vi "SVFA FFT Spectrum (Real-Im) (1 Ch).vi"(0 "scaled signal [EU]":waveform(dbl), 2 "window":T9=1 items=["None"=0, "Hanning"=1, "Hamming"=2, "Blackman-Harris"=3, "Exact Blackman"=4, "Blackman"=5, "Flat Top"=6, "4 Term B-Harris "=7, "7 Term B-Harris"=8, "Low Sidelobe"=9, "Force"=64, "Exponential"=65, "Blackman Nuttall"=11, "Triangle"=30, "Bartlett-Hanning"=31, "Bohman"=32, "Parzen"=33, "Welch"=34, "Kaiser"=60, "Dolph-Chebyshev"=61, "Gaussian"=62], 5 "error in (no error)":errorcluster, 7 "averaging parameters":T7={"averaging mode"=enum."No averaging", "weighting mode"=enum."Exponential", "number of averages"=10, "linear mode"=enum."One shot"} {"number of averages" min=1 step=1}, 9 "restart averaging (F)":bool) -> (11 "averaging done":bool, 13 "averages completed":dbl, 14 "real part [EU rms]":cluster{"f0":dbl, "df":dbl, "real part":dbl[]} {"real part" format="%.2f"; "df" format="%.2f"; "f0" format="%.2f"}, 16 "imaginary part [EU rms]":T8 {"imaginary part" format="%.2f"; "df" format="%.2f"; "f0" format="%.2f"}, 17 "unit label":string, 18 "spectrum info":T1={"channel name"="", "description"="", "x-axis units"=0, "spectral info"={"spectrum type"=enum."Power [Magnitude^2]", "linear/dB"=enum."linear", "window"=0, "window size"=0, "FFT size"=0}, "engineering units"=0, "custom label"="", "dB reference [EU]"=0.0, "peak units"=enum."rms", "weighting filter"=0, "spectral density?"=FALSE, "unit label"="", "spectrum skewed?"=FALSE, "complimentary spectrum units"=enum."none"} {"x-axis units" items=["Time (s)"=0, "Frequency-CB (Hz)"=1, "Frequency-CPB (Hz)"=1248, "Frequency-Arbitrary (Hz)"=2357, "Quefrency (s)"=2, "Revolutions (rev)"=3, "Order"=4, "Speed (RPM)"=11, "Speed (rad/s)"=21, "Index"=65535]; "weighting filter" items=["Linear", "A-weighting", "B-weighting", "C-weighting", "ITU-R 468-4", "Dolby", "CCITT", "C-message", "Wb", "Wc", "Wd", "We", "Wf", "Wh", "Wj", "Wk", "Wm", "AES17 20 kHz lowpass", "AES17 40 kHz lowpass", "AES17 20 kHz highpass", "AES17 40 kHz highpass"]; "dB reference [EU]" format="%.2f"; "engineering units" items=["custom..."=0, "V"=1, "A"=21, "C"=30, "pC"=31, "s"=32, "-"=29, "Pa"=2, "N"=20, "g"=3, "m/s^2"=4, "m/s"=5, "m"=6, "mm/s"=12, "mm"=13, "micron/s"=14, "micron"=15, "in/s^2"=7, "in/s"=8, "in"=9, "mil/s"=10, "mil"=11, "rad/s^2"=16, "rad/s"=17, "rad"=18, "deg/s^2"=26, "deg/s"=27, "deg"=28, "RPM"=22, "cycle/s^2"=23, "Hz"=24, "cycle"=25, "strain"=19]; "spectral info"."window" items=["None "=0, "Hanning"=1, "Hamming"=2, "Blackman-Harris"=3, "Exact Blackman"=4, "Blackman"=5, "Flat Top"=6, "4 Term B-Harris "=7, "7 Term B-Harris"=8, "Low Sidelobe"=9, "Force - Exponential"=10, "Gaussian"=62]}, 19 "error out":errorcluster)   [LabVIEW 2017]
doc: "Computes the Fast Fourier Transform (FFT) spectrum of <B>scaled signal [EU]</B>. This VI returns FFT results as the real and imaginary parts, or the first and second elements of the ordered pairs, of the FFT spectrum. Wire data to the <B>scaled signal [EU]</B> input to determine the polymorphic instance to use or manually select the instance."
uses:
  <vilib>/addons/_NISVFA/_Shared subVIs/Controls/svc_Window.ctl
  <vilib>/addons/_NISVFA/_Shared subVIs/Controls/svc_Spectrum Info.ctl
  <vilib>/addons/_NISVFA/_Shared subVIs/Controls/svc_X-Axis Units.ctl
  <vilib>/addons/_NISVFA/_Shared subVIs/Controls/svc_Spectrum Type.ctl
  <vilib>/addons/_NISVFA/_Shared subVIs/Controls/svc_Engineering Units Text Ring.ctl
  <vilib>/addons/_NISVFA/_Shared subVIs/Controls/svc_Weighting Filter Text Ring.ctl
  <vilib>/addons/_NISVFA/_Shared subVIs/Controls/svc_Complimentary Spectrum Units.ctl
  <vilib>/Analysis/2dsp.llb/Real FFT.vi
  <vilib>/Analysis/2dsp.llb/Power Spectrum (DBL).vi
  <vilib>/addons/_NISVFA/_Shared subVIs/Windowing/svfa_Scaled Time Domain Window (Array).vi
  <vilib>/addons/_NISVFA/_Shared subVIs/Common/svc_Get SV Channel Info.vi
  <vilib>/addons/_NISVFA/_Shared subVIs/Common/svc_Spectrum Units.vi
  <vilib>/addons/_NISVFA/_Shared subVIs/Spectrum Averaging/svfa_No Average Array (complex).vi
  <vilib>/addons/_NISVFA/_Shared subVIs/Spectrum Averaging/svfa_Average Array (complex).vi
  <vilib>/addons/_NISVFA/_Shared subVIs/Spectrum Averaging/svfa_No Average Array (real).vi
  <vilib>/addons/_NISVFA/_Shared subVIs/Spectrum Averaging/svfa_Average Array (real).vi
  <vilib>/addons/_NISVFA/_Shared subVIs/Spectrum Averaging/svfa_Peak Hold Array.vi
  <vilib>/Analysis/4window.llb/Force Window.vi
  <vilib>/Analysis/4window.llb/Force Window (DBL).vi
  <vilib>/Analysis/4window.llb/Exponential Window.vi
  <vilib>/Analysis/4window.llb/Exponential Window (DBL).vi
  <vilib>/Utility/error.llb/Error Cluster From Error Code.vi
  <vilib>/Analysis/0measdsp.llb/Scaled Time Domain Window.vi
  <vilib>/Analysis/0measdsp.llb/Scaled Time Domain Window (DBL).vi
  <vilib>/addons/_NISVFA/_Spectrum Processing/subVIs/svfa_Spectrum Info Window to windowTd Type Def.vi
  <vilib>/addons/_NISVFA/_Shared subVIs/Common/svc_Window Parameters.vi
  <vilib>/addons/_NISVFA/_Shared subVIs/Common/svc_Get Window Info.vi
  <vilib>/addons/_NISVFA/_Shared subVIs/Common/svc_Get Weighting Enum and Labels.vi
  <vilib>/addons/_NISVFA/_Shared subVIs/Common/svc_Unit Label Lexical Class.vi
  <vilib>/addons/_NISVFA/_Shared subVIs/Common/svc_Engineering Units to Unit Label.vi
  <vilib>/addons/_NISVFA/_Shared subVIs/Common/svc_Format Value (DBL).vi
  <vilib>/addons/_NISVFA/_Shared subVIs/Common/svc_Channel Info to Spectrum Info.vi
  <vilib>/addons/_NISVFA/_Shared subVIs/Common/svc_Unit Label to Engineering Units.vi
  <vilib>/Analysis/NI_AALPro.lvlib
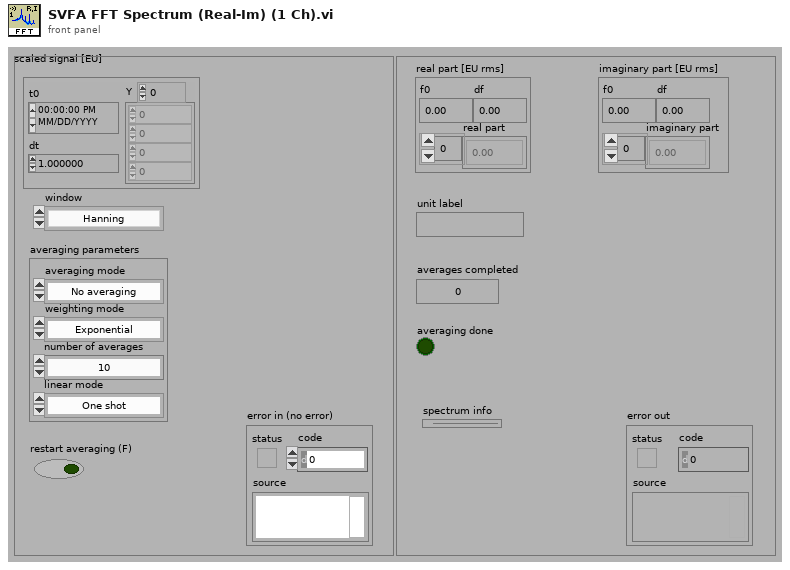
[diagram p1: front panel]
types:
  T1 = typedef "svc_Spectrum Info.ctl" = cluster{"channel name":string, "description":string, "x-axis units":T2, "spectral info":cluster{"spectrum type":T3, "linear/dB":enum16{"linear", "dB"}, "window":u16, "window size":i32, "FFT size":i32}, "engineering units":T4, "custom label":string, "dB reference [EU]":dbl, "peak units":enum16{"rms", "peak", "peak-peak"}, "weighting filter":T5, "spectral density?":bool, "unit label":string, "spectrum skewed?":bool, "complimentary spectrum units":T6}
  T2 = typedef "svc_X-Axis Units.ctl" = u16
  T3 = typedef "svc_Spectrum Type.ctl" = enum16{"FFT Spectrum [complex]", "Amplitude [Magnitude]", "Power [Magnitude^2]", "Cross Spectrum [complex]", "Frequency Response [Complex]"}
  T4 = typedef "svc_Engineering Units Text Ring.ctl" = u16
  T5 = typedef "svc_Weighting Filter Text Ring.ctl" = u16
  T6 = typedef "svc_Complimentary Spectrum Units.ctl" = enum16{"none", "radians", "degrees", "cycles", "imaginary"}
  T7 = cluster{"averaging mode":enum16{"No averaging", "Vector averaging", "RMS averaging", "Peak hold"}, "weighting mode":enum16{"Linear", "Exponential"}, "number of averages":u32, "linear mode":enum16{"One shot", "Auto restart"}}
  T8 = cluster{"f0":dbl, "df":dbl, "imaginary part":dbl[]}
  T9 = typedef "svc_Window.ctl" = u32
  T10 = cluster{"f0":dbl, "df":dbl, "complex spectrum":cdb[]}
  T11 = enum16{"Restart processing", "Continue processing", "Skip processing"}
  T12 = enum16{"No averaging", "Vector averaging", "RMS averaging", "Peak hold"}
  T13 = cluster{"complex FFT":cdb[], "real FFT":dbl[], "f0":dbl, "df":dbl, "averages completed":dbl, "averaging parameters":cluster{"averaging mode":enum16{"No averaging", "Vector averaging", "RMS averaging", "Peak hold"}, "weighting mode":enum16{"Linear", "Exponential"}, "number of averages":u32, "linear mode":enum16{"One shot", "Auto restart"}}}
  T14 = cluster{"complex FFT":cdb[], "Mag/Real FFT":dbl[], "f0":dbl, "df":dbl, "averages completed":dbl, "averaging parameters":cluster{"averaging mode":enum16{"No averaging", "Vector averaging", "RMS averaging", "Peak hold"}, "weighting mode":enum16{"Linear", "Exponential"}, "number of averages":u32, "linear mode":enum16{"One shot", "Auto restart"}}}
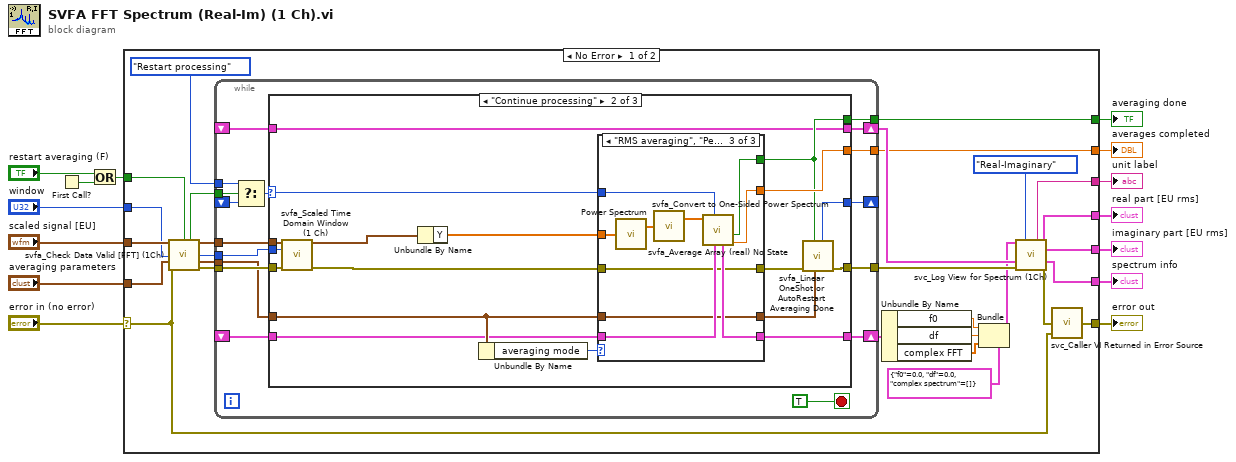
[diagram p0: block diagram]
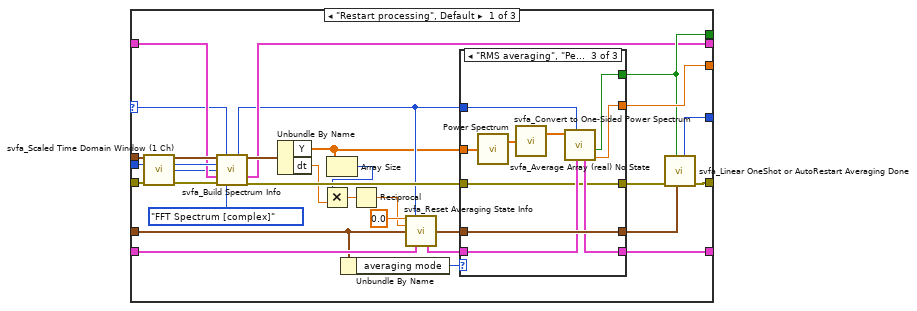
[diagram p2: hidden frame]
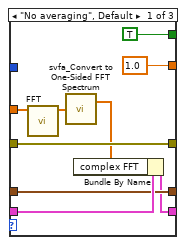
[diagram p3: hidden frame]
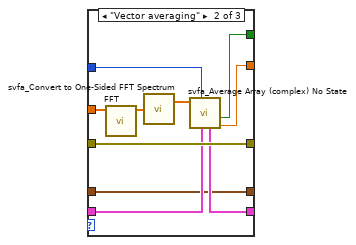
[diagram p4: hidden frame]
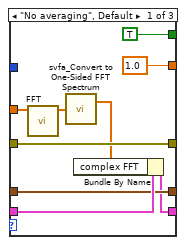
[diagram p5: hidden frame]
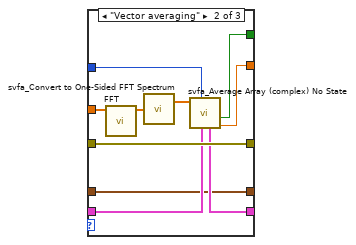
[diagram p6: hidden frame]
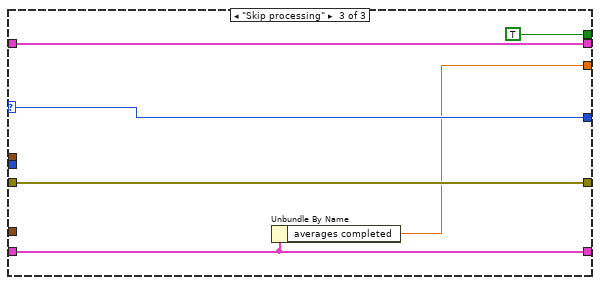
[diagram p7: hidden frame]
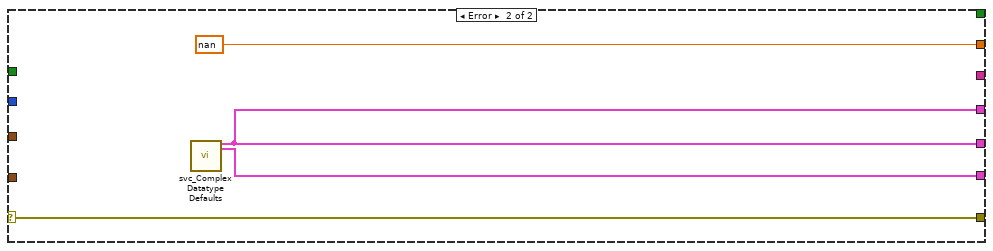
[diagram p8: hidden frame]
diagram:
  n1 = First Call?() -> (First Call?: T/F=w3:bool)
  n2 = Or(x="restart averaging (F)", y=w3) -> (x .or. y?=w1:bool)
  n3 = case shown="No Error" "error in (no error)" {
    selector: "error in (no error)" -> [w30 w177]
    tunnel: "window" -> [w35 _]
    tunnel: "averaging parameters" -> [w34 _]
    tunnel: [w33 w177] -> w14
    tunnel: [w39 _] -> w13
    tunnel: "scaled signal [EU]" -> [w42 _]
    tunnel: w1 -> [w40 _]
    tunnel: [w16 nan ("averages completed")] -> w8
    tunnel: [w17 _] -> w7
    tunnel: [w36 w174] -> w4
    tunnel: [w38 w175] -> w6
    tunnel: [w37 w175] -> w5
    frame No Error {
      n4 = call <vilib>:"svfa_Check Data Valid [FFT] (1Ch).vi"("signal in [X]"=w42, "restart averaging (F)"=w40, "window"=w35, "averaging parameters"=w34, "error in (no error)"=w30) -> ("restart averaging"=w25:bool, "dup signal in [X]"=w29:waveform(dbl), "dup window"=w28:T9, "dup averaging parameters"=w27:T7, "error out"=w26:errorcluster)  [unwired: 6 in]
      n5 = while {
        shift-left: _ -> [w51]
        shift-right: [w52] -> w31
        tunnel: [w54] -> w22
        tunnel: w25 -> [w49]
        tunnel: w26 -> [w55]
        tunnel: w29 -> [w56]
        tunnel: [w57] -> w17
        tunnel: [w59] -> w16
        shift-right: [w58] -> _
        shift-left: _ -> [w48]
        shift-right: [w50] -> w23
        shift-left: _ -> [w46]
        tunnel: T11."Restart processing" ("t") -> [w45]
        tunnel: w27 -> [w44]
        tunnel: w28 -> [w43]
        stop <- TRUE stop-if-true
        n6 = Select(t=w45, s=w49, f=w48) -> (s? t:f=w47:T11)
        n7 = case shown="\"Continue processing\"" w47 {
          selector: w47 -> [w73 w123 w173]
          tunnel: [w90 w137 w170] -> w59
          tunnel: [w76 w129 w169] -> w52
          tunnel: [w89 w136 w173] -> w58
          tunnel: [w88 w135 TRUE ("averaging done")] -> w57
          tunnel: w44 -> [w66 w122 _]
          tunnel: w56 -> [w87 w134 _]
          tunnel: w55 -> [w74 w128 w172]
          tunnel: w43 -> [w83 w133 _]
          tunnel: [w81 w131 w172] -> w54
          tunnel: w51 -> [w71 w121 w169]
          tunnel: [w78 w124 w168] -> w50
          tunnel: w46 -> [w77 w124 w168]
          frame "Restart processing", Default {
            n8 = call <vilib>:"svfa_Scaled Time Domain Window (1 Ch).vi"("Signal in [X]"=w87, "window"=w83, "error in"=w74) -> ("Windowed Waveform"=w84:waveform(dbl), "dup window"=w80:T9, "window length"=w63:i32, "error out"=w86:errorcluster)  [unwired: 7 in, 2 out]
            n9 = call <vilib>:"svfa_Build Spectrum Info.vi"("scaled signal [EU]"=w84, "processing control"=w73, "window"=w80, "window size"=w63, "spectrum info in"=w77, "error in (no error)"=w86, "spectrum type"=svc_Spectrum_Type."FFT Spectrum [complex]") -> ("dup processing control"=w62:T11, "dup scaled signal [EU]"=w79:waveform(dbl), "spectrum info out"=w78:T1, "error out"=w85:errorcluster)  [unwired: 5 in]
            n10 = Unbundle By Name ("Get Waveform Components")(w79) -> ("Y"=w61:dbl[], "dt"=w64:dbl)
            n11 = Array Size(array=w61) -> (size(s)=w60:i32)
            n12 = Multiply(x=w60, y=w64) -> (x*y=w72:dbl)
            n13 = Unbundle By Name(w66) -> ("averaging mode"=w91:T12)
            n14 = Reciprocal(x=w72) -> (1/x=w65:dbl)
            n15 = call <vilib>:"svfa_Reset Averaging State Info.vi"("f0"=0.0, "processing control"=w62, "df"=w65, "averaging parameters"=w66, "averaging state info in"=w71) -> ("dup averaging parameters"=w69:T7, "averaging state info out"=w70:T13)  [unwired: 9 in]
            n16 = case shown="\"RMS averaging\", \"Peak hold\"" w91 {
              tunnel: [w98 w107 w111] -> w82
              tunnel: [TRUE ("averaging done") w101 w116] -> w88
              tunnel: [1.0 ("averages completed") w102 w115] -> w90
              tunnel: w61 -> [w95 w109 w119]
              tunnel: w85 -> [w98 w107 w111]
              tunnel: w62 -> [_ w103 w114]
              tunnel: [w92 w105 w112] -> w76
              tunnel: w70 -> [w97 w106 w113]
              tunnel: w69 -> [w93 w104 w117]
              tunnel: [w93 w104 w117] -> w68
              frame "No averaging", Default {
                n17 = call-poly <vilib>:"FFT.vi"("X"=w95) -> ("FFT {X}"=w96:cdb[])  [unwired: 9 in, 1 out]
                n18 = call <vilib>:"svfa_Convert to One-Sided FFT Spectrum.vi"("two-sided FFT spectrum"=w96) -> ("one-sided FFT spectrum"=w94:cdb[])  [unwired: 1 out]
                n19 = Bundle By Name(cluster=w97, "complex FFT"=w94) -> (w92:T13)
              }
              frame "Vector averaging" {
                n20 = call-poly <vilib>:"FFT.vi"("X"=w109) -> ("FFT {X}"=w110:cdb[])  [unwired: 9 in, 1 out]
                n21 = call <vilib>:"svfa_Convert to One-Sided FFT Spectrum.vi"("two-sided FFT spectrum"=w110) -> ("one-sided FFT spectrum"=w108:cdb[])  [unwired: 1 out]
                n22 = call <vilib>:"svfa_Average Array (complex) No State.vi"("averaging state info in"=w106, "processing control"=w103, "array"=w108) -> ("averages completed"=w102:dbl, "averaging done"=w101:bool, "averaging state info out"=w105:T14)  [unwired: 5 in, 1 out]
              }
              frame "RMS averaging", "Peak hold" {
                n23 = call-poly <vilib>:"Power Spectrum.vi"("X"=w119) -> ("Power Spectrum"=w120:dbl[])  [unwired: 1 out]
                n24 = call <vilib>:"svfa_Convert to One-Sided Power Spectrum.vi"("two-sided power spectrum"=w120) -> ("one-sided power spectrum"=w118:dbl[])  [unwired: 1 out]
                n25 = call <vilib>:"svfa_Average Array (real) No State.vi"("averaging state info in"=w113, "processing control"=w114, "array"=w118) -> ("averages completed"=w115:dbl, "averaging done"=w116:bool, "averaging state info out"=w112:T14)  [unwired: 5 in, 1 out]
              }
            }
            n26 = call <vilib>:"svfa_Linear OneShot or AutoRestart Averaging Done.vi"("averaging parameters"=w68, "averaging done"=w88, "error in (no error)"=w82) -> ("error out"=w81:errorcluster, "processing control"=w89:T11)  [unwired: 7 in]
          }
          frame "Continue processing" {
            n27 = call <vilib>:"svfa_Scaled Time Domain Window (1 Ch).vi"("Signal in [X]"=w134, "window"=w133, "error in"=w128) -> ("Windowed Waveform"=w125:waveform(dbl), "error out"=w126:errorcluster)  [unwired: 7 in, 4 out]
            n28 = Unbundle By Name ("Get Waveform Components")(w125) -> ("Y"=w130:dbl[])
            n29 = Unbundle By Name(w122) -> ("averaging mode"=w138:T12)
            n30 = case shown="\"RMS averaging\", \"Peak hold\"" w138 {
              tunnel: [w145 w154 w159] -> w132
              tunnel: [TRUE ("averaging done") w148 w164] -> w135
              tunnel: [1.0 ("averages completed") w149 w163] -> w137
              tunnel: w130 -> [w142 w156 w166]
              tunnel: w126 -> [w145 w154 w159]
              tunnel: w123 -> [_ w150 w162]
              tunnel: [w139 w152 w160] -> w129
              tunnel: w121 -> [w144 w153 w161]
              tunnel: w122 -> [w140 w151 w158]
              tunnel: [w140 w151 w158] -> w127
              frame "No averaging", Default {
                n31 = call-poly <vilib>:"FFT.vi"("X"=w142) -> ("FFT {X}"=w143:cdb[])  [unwired: 9 in, 1 out]
                n32 = call <vilib>:"svfa_Convert to One-Sided FFT Spectrum.vi"("two-sided FFT spectrum"=w143) -> ("one-sided FFT spectrum"=w141:cdb[])  [unwired: 1 out]
                n33 = Bundle By Name(cluster=w144, "complex FFT"=w141) -> (w139:T14)
              }
              frame "Vector averaging" {
                n34 = call-poly <vilib>:"FFT.vi"("X"=w156) -> ("FFT {X}"=w157:cdb[])  [unwired: 9 in, 1 out]
                n35 = call <vilib>:"svfa_Convert to One-Sided FFT Spectrum.vi"("two-sided FFT spectrum"=w157) -> ("one-sided FFT spectrum"=w155:cdb[])  [unwired: 1 out]
                n36 = call <vilib>:"svfa_Average Array (complex) No State.vi"("averaging state info in"=w153, "processing control"=w150, "array"=w155) -> ("averages completed"=w149:dbl, "averaging done"=w148:bool, "averaging state info out"=w152:T14)  [unwired: 5 in, 1 out]
              }
              frame "RMS averaging", "Peak hold" {
                n37 = call-poly <vilib>:"Power Spectrum.vi"("X"=w166) -> ("Power Spectrum"=w167:dbl[])  [unwired: 1 out]
                n38 = call <vilib>:"svfa_Convert to One-Sided Power Spectrum.vi"("two-sided power spectrum"=w167) -> ("one-sided power spectrum"=w165:dbl[])  [unwired: 1 out]
                n39 = call <vilib>:"svfa_Average Array (real) No State.vi"("averaging state info in"=w161, "processing control"=w162, "array"=w165) -> ("averages completed"=w163:dbl, "averaging done"=w164:bool, "averaging state info out"=w160:T14)  [unwired: 5 in, 1 out]
              }
            }
            n40 = call <vilib>:"svfa_Linear OneShot or AutoRestart Averaging Done.vi"("averaging parameters"=w127, "averaging done"=w135, "error in (no error)"=w132) -> ("error out"=w131:errorcluster, "processing control"=w136:T11)  [unwired: 7 in]
          }
          frame "Skip processing" {
            n41 = Unbundle By Name(w169) -> ("averages completed"=w170:dbl)
          }
        }
      }
      n42 = Unbundle By Name(w31) -> ("f0"=w21:dbl, "df"=w20:dbl, "complex FFT"=w19:cdb[])
      n43 = Bundle(cluster=T10 {"f0"=0.0, "df"=0.0, "complex spectrum"=[]} ("complex spectrum response"), "f0"=w21, "df"=w20, "complex spectrum"=w19) -> (w18:T10)
      n44 = call <vilib>:"svc_Log View for Spectrum (1Ch).vi"("complex spectrum"=w18, "View"=enum16{"Mag-Phase", "Real-Imaginary"}."Real-Imaginary", "spectrum info in"=w23, "error in (no error)"=w22) -> ("unit label [mag or real]"=w39:string, "magnitude or real"=w38:cluster{"f0":dbl, "df":dbl, dbl[]}, "phase or imag"=w37:cluster{"f0":dbl, "df":dbl, dbl[]}, "spectrum info out"=w36:T1, "error out"=w41:errorcluster)  [unwired: 6 in, 1 out]
      n45 = call <vilib>:"svc_Caller VI Returned in Error Source.vi"("warning input to caller"=w30, "error in (no error)"=w41) -> ("error out"=w33:errorcluster)  [unwired: 3 in]
    }
    frame Error {
      n46 = call <vilib>:"svc_Complex Datatype Defaults.vi"() -> ("empty spectrum"=w175:cluster{"f0":dbl, "df":dbl, "magnitude":dbl[]}, "dead spectrum info"=w174:T1)  [unwired: 11 in, 7 out]
    }
  }
  "error out" <- w14
  "real part [EU rms]" <- w6
  "imaginary part [EU rms]" <- w5
  "unit label" <- w13
  "averages completed" <- w8
  "averaging done" <- w7
  "spectrum info" <- w4
